vi "Perform Action.vi"(8 "error in":errorcluster, 10 "Input":variant, 11 "Virt Instrument Base in":refnum<class "Virt Instr Target Linear Scale.lvclass">) -> (0 "error out":errorcluster, 2 "Output":variant, 3 "Virt Instrument Base out":refnum<class "Virt Instr Target Linear Scale.lvclass">)   [LabVIEW 2023, in "HAL GOOP4.lvlib" / "Virt Instr Target Linear Scale.lvclass"]
uses:
  Virt Instr Target Linear Scale.lvclass
  D:/git/HAL/HAL GOOP4/Virt Instr Base/Virt Instr Base.lvclass
  Virt Instr Base/Virt Instr Base.lvclass/Virt Instr Base.ctl
  2c2c3eeb-15f5-4b0f-81a3-0cbafe2fdac7.vi
  <vilib>/JDP Science/JSONtext/JSON text to Variant.vi
  Virt Instr Target/Virt Instr Target.lvclass
  <vilib>/JDP Science/JSONtext/LVClass Serializer/JSONtext LVClass Serializer.lvclass
  Virt Instr Target Linear Scale.lvclass/Virt Instr Target Linear Scale.ctl
  <userlib>/_OpenG.lib/lvdata/lvdata.llb/openg_variant.lvlib
  Virt Instr Base/Virt Instr Base.lvclass
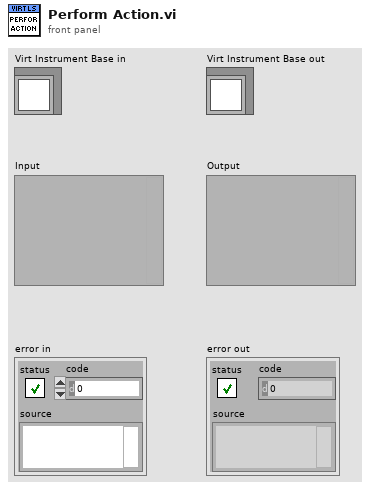
[diagram p1: front panel]
types:
  T1 = cluster{"Input min":dbl, "Input max":dbl, "Output min":dbl, "Output max":dbl}
  T2 = typedef "openg_variant.lvlib/Type Descriptor Enumeration__ogtk.ctl" = enum8{"<Null>", "I8", "I16", "I32", "I64", "U8", "U16", "U32", "U64", "SGL", "DBL", "EXT", "CSG", "CDB", "CXT", "0x0F", "0x10", "0x11", "0x12", "0x13", "0x14", "Enum U8", "Enum U16", "Enum U32", "Enum U64", "SGL PQ", "DBL PQ", "EXT PQ", "CSG PQ", "CDB PQ", "CXT PQ", "0x1F", "0x20", "Boolean", "0x22", "0x23", "0x24", "0x25", "0x26", "0x27", "0x28", "0x29", "0x2A", "0x2B", "0x2C", "0x2D", "0x2E", "0x2F", "String", "0x31", "Path", "Pict", "0x34", "0x35", "0x36", "DAQ", "0x38", "0x39", "0x3A", "0x3B", "0x3C", "0x3D", "0x3E", "0x3F", "Array", "0x41", "0x42", "0x43", "0x44", "0x45", "0x46", "0x47", "0x48", "0x49", "0x4A", "0x4B", "0x4C", "0x4D", "0x4E", "0x4F", "Cluster", "0x51", "0x52", "Variant", "Waveform", "0x55", "0x56", "0x57", "0x58", "0x59", "0x5A", "0x5B", "0x5C", "0x5D", "0x5E", "Fixed Point", "0x60", "0x61", "0x62", "0x63", "0x64", "0x65", "0x66", "0x67", "0x68", "0x69", "0x6A", "0x6B", "0x6C", "0x6D", "0x6E", "0x6F", "Refnum", "0x71", "0x72", "Set Collection", "Map Collection"}
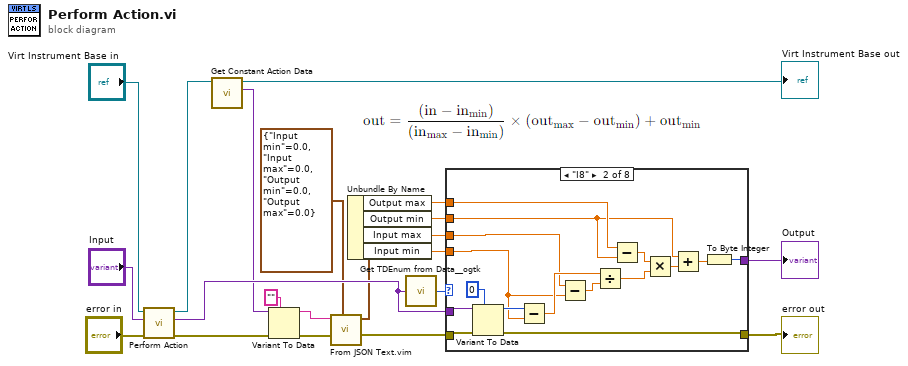
[diagram p0: block diagram]
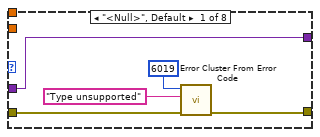
[diagram p2: hidden frame]
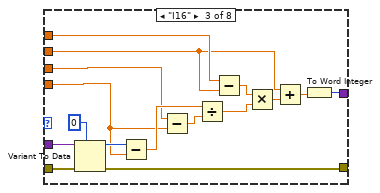
[diagram p3: hidden frame]
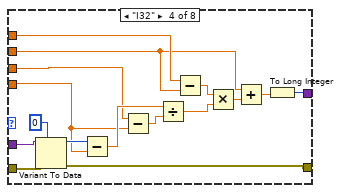
[diagram p4: hidden frame]
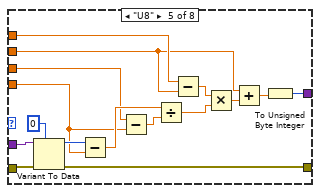
[diagram p5: hidden frame]
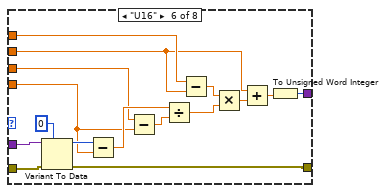
[diagram p6: hidden frame]
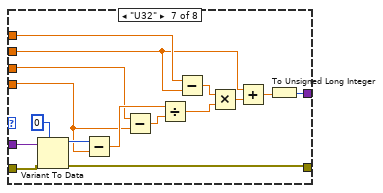
[diagram p7: hidden frame]
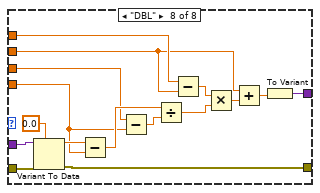
[diagram p8: hidden frame]
diagram:
  n1 = call-parent "Perform Action.vi"("error in"="error in", "Input"="Input", "Virt Instrument Base in"="Virt Instrument Base in") -> ("error out"=w17:errorcluster, "Output"=w12:variant, "Virt Instrument Base out"=w14:refnum<class "Virt Instr Target Linear Scale.lvclass">)  [unwired: 6 in]
  n2 = call "Get Constant Action Data.vi"("Virt Instr Base in"=w14) -> ("Constant Action Data"=w7:variant, "Virt Instr Base out"=→"Virt Instrument Base out":refnum<class "Virt Instr Target Linear Scale.lvclass">)  [unwired: 9 in]
  n3 = Variant To Data(error in=w17, type="", Variant=w7) -> (data=w8:string, error out=w10:errorcluster)
  n4 = call "From JSON Text.vim"("Data Type and Default Value"=T1 {"Input min"=0.0, "Input max"=0.0, "Output min"=0.0, "Output max"=0.0}, "error in (no error)"=w10, "JSON"=w8) -> ("error out"=w9:errorcluster, "Data out"=w5:T1)  [unwired: 7 in]
  n5 = Unbundle By Name(w5) -> ("Output max"=w2:dbl, "Output min"=w1:dbl, "Input max"=w3:dbl, "Input min"=w4:dbl)
  n6 = call <userlib>:"Get TDEnum from Data__ogtk.vi"("Data"=w12) -> ("Type Descriptor Enumeration"=w18:T2)  [unwired: 4 in]
  n7 = case shown="\"I8\"" w18 {
    tunnel: w9 -> [w26 w33 w44 w66 w77 w93 w110 w136]
    tunnel: w12 -> [w25 w32 w45 w65 w78 w94 w109 w135]
    tunnel: [w24 w27 w43 w59 w75 w91 w107 w134] -> w16
    tunnel: [w25 w34 w50 w60 w76 w92 w108 w133] -> w15
    tunnel: w4 -> [_ w28 w46 w61 w79 w95 w111 w130]
    tunnel: w3 -> [_ w29 w47 w62 w80 w96 w112 w131]
    tunnel: w2 -> [_ w31 w49 w64 w82 w98 w114 w128]
    tunnel: w1 -> [_ w30 w48 w63 w81 w97 w113 w124]
    frame "<Null>", Default {
      n8 = call <vilib>:"Error Cluster From Error Code.vi"("error in (no error)"=w26, "error message (\"\")"="Type unsupported" ("error message (\"\")"), "error code (0)"=6019) -> ("error out"=w24:errorcluster)  [unwired: 6 in]
    }
    frame "I8" {
      n9 = Variant To Data(error in=w33, type=i8 0, Variant=w32) -> (data=w41:i8, error out=w27:errorcluster)
      n10 = Subtract(x=w41, y=w28) -> (x-y=w40:dbl)
      n11 = Subtract(x=w29, y=w28) -> (x-y=w39:dbl)
      n12 = Divide(x=w40, y=w39) -> (x/y=w37:dbl)
      n13 = Subtract(x=w31, y=w30) -> (x-y=w38:dbl)
      n14 = Multiply(x=w38, y=w37) -> (x*y=w36:dbl)
      n15 = Add(x=w30, y=w36) -> (x+y=w35:dbl)
      n16 = To Byte Integer(number=w35) -> (8bit integer=w34:i8)
    }
    frame "I16" {
      n17 = Variant To Data(error in=w44, type=i16 0, Variant=w45) -> (data=w57:i16, error out=w43:errorcluster)
      n18 = Subtract(x=w57, y=w46) -> (x-y=w56:dbl)
      n19 = Subtract(x=w47, y=w46) -> (x-y=w55:dbl)
      n20 = Divide(x=w56, y=w55) -> (x/y=w53:dbl)
      n21 = Subtract(x=w49, y=w48) -> (x-y=w54:dbl)
      n22 = Multiply(x=w54, y=w53) -> (x*y=w52:dbl)
      n23 = Add(x=w48, y=w52) -> (x+y=w51:dbl)
      n24 = To Word Integer(number=w51) -> (16bit integer=w50:i16)
    }
    frame "I32" {
      n25 = Variant To Data(error in=w66, type=0, Variant=w65) -> (data=w73:i32, error out=w59:errorcluster)
      n26 = Subtract(x=w73, y=w61) -> (x-y=w72:dbl)
      n27 = Subtract(x=w62, y=w61) -> (x-y=w71:dbl)
      n28 = Divide(x=w72, y=w71) -> (x/y=w69:dbl)
      n29 = Subtract(x=w64, y=w63) -> (x-y=w70:dbl)
      n30 = Multiply(x=w70, y=w69) -> (x*y=w68:dbl)
      n31 = Add(x=w63, y=w68) -> (x+y=w67:dbl)
      n32 = To Long Integer(number=w67) -> (32bit integer=w60:i32)
    }
    frame "U8" {
      n33 = Variant To Data(error in=w77, type=u8 0, Variant=w78) -> (data=w89:u8, error out=w75:errorcluster)
      n34 = Subtract(x=w89, y=w79) -> (x-y=w88:dbl)
      n35 = Subtract(x=w80, y=w79) -> (x-y=w87:dbl)
      n36 = Divide(x=w88, y=w87) -> (x/y=w85:dbl)
      n37 = Subtract(x=w82, y=w81) -> (x-y=w86:dbl)
      n38 = Multiply(x=w86, y=w85) -> (x*y=w84:dbl)
      n39 = Add(x=w81, y=w84) -> (x+y=w83:dbl)
      n40 = To Unsigned Byte Integer(number=w83) -> (unsigned 8bit integer=w76:u8)
    }
    frame "U16" {
      n41 = Variant To Data(error in=w93, type=u16 0, Variant=w94) -> (data=w105:u16, error out=w91:errorcluster)
      n42 = Subtract(x=w105, y=w95) -> (x-y=w104:dbl)
      n43 = Subtract(x=w96, y=w95) -> (x-y=w103:dbl)
      n44 = Divide(x=w104, y=w103) -> (x/y=w101:dbl)
      n45 = Subtract(x=w98, y=w97) -> (x-y=w102:dbl)
      n46 = Multiply(x=w102, y=w101) -> (x*y=w100:dbl)
      n47 = Add(x=w97, y=w100) -> (x+y=w99:dbl)
      n48 = To Unsigned Word Integer(number=w99) -> (unsigned 16bit integer=w92:u16)
    }
    frame "U32" {
      n49 = Variant To Data(error in=w110, type=u32 0, Variant=w109) -> (data=w121:u32, error out=w107:errorcluster)
      n50 = Subtract(x=w121, y=w111) -> (x-y=w120:dbl)
      n51 = Subtract(x=w112, y=w111) -> (x-y=w119:dbl)
      n52 = Divide(x=w120, y=w119) -> (x/y=w117:dbl)
      n53 = Subtract(x=w114, y=w113) -> (x-y=w118:dbl)
      n54 = Multiply(x=w118, y=w117) -> (x*y=w116:dbl)
      n55 = Add(x=w113, y=w116) -> (x+y=w115:dbl)
      n56 = To Unsigned Long Integer(number=w115) -> (unsigned 32bit integer=w108:u32)
    }
    frame "DBL" {
      n57 = Variant To Data(error in=w136, type=0.0, Variant=w135) -> (data=w137:dbl, error out=w134:errorcluster)
      n58 = Subtract(x=w137, y=w130) -> (x-y=w132:dbl)
      n59 = Subtract(x=w131, y=w130) -> (x-y=w129:dbl)
      n60 = Divide(x=w132, y=w129) -> (x/y=w126:dbl)
      n61 = Subtract(x=w128, y=w124) -> (x-y=w127:dbl)
      n62 = Multiply(x=w127, y=w126) -> (x*y=w125:dbl)
      n63 = Add(x=w124, y=w125) -> (x+y=w123:dbl)
      n64 = To Variant(anything=w123) -> (Variant=w133:variant)
    }
  }
  "error out" <- w16
  "Output" <- w15
